vi "GET list step count.vi"(7 "Message":refnum<class "API Message.lvclass">, 8 "error in (no error)":errorcluster, 11 "API Message in":refnum<class "API Message.lvclass">) -> (0 "error out":errorcluster, 3 "API Message out":refnum<class "API Message.lvclass">)   [LabVIEW 2017]
uses:
  Response/Response.lvclass
  API Message.lvclass
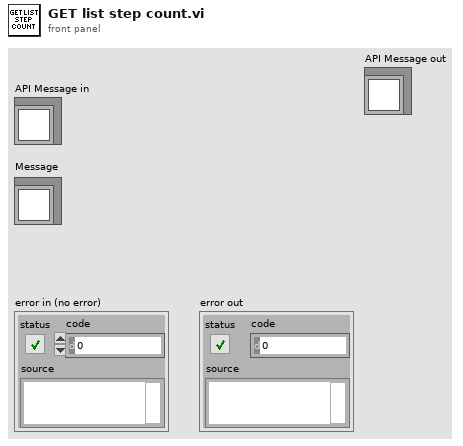
[diagram p1: front panel]
types:
  T1 = cluster{"error":bool, "message":string, "count":u32}
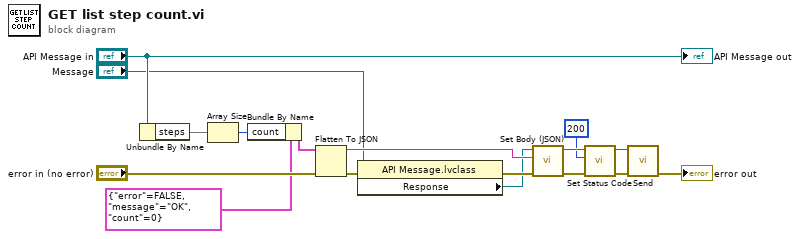
[diagram p0: block diagram]
diagram:
  n1 = Unbundle By Name("API Message in") -> ("steps"=w2)
  n2 = Array Size(array=w2) -> (size(s)=w1:i32)
  n3 = Bundle By Name(cluster=T1 {"error"=FALSE, "message"="OK", "count"=0}, "count"=w1) -> (w13:T1)
  n4 = Flatten To JSON(anything=w13, error in (no error)="error in (no error)") -> (JSON string=w12:string, 11:w11:errorcluster)  [unwired: 1 in]
  n5 = property class="API Message.lvclass"(reference="Message", error in=w11) -> (error out=w5:errorcluster, "Response"=w3:refnum<class "Response.lvclass">)  [unwired: 1 out]
  n6 = call "Set Body (JSON).vi"("error in (no error)"=w5, "Header"=w12, "Response in"=w3) -> ("error out"=w9:errorcluster, "Response out"=w10:refnum<class "Response.lvclass">)  [unwired: 7 in]
  n7 = call "Set Status Code.vi"("error in (no error)"=w9, "Status Code"=u16 200, "Response in"=w10) -> ("error out"=w7:errorcluster, "Response out"=w6:refnum<class "Response.lvclass">)  [unwired: 7 in]
  n8 = call "Send.vi"("error in (no error)"=w7, "Response in"=w6) -> ("error out"=→"error out":errorcluster)  [unwired: 9 in]
  "API Message out" <- "API Message in"
